vi "Read Msg Output.vi"(11 "TEMPLATE Msg Output in":refnum<class "TEMPLATE Msg Output.lvclass">) -> ()   [LabVIEW 2020, in "_Template.lvlib" / "Templates.lvlib" / "TEMPLATE jettl Msg.lvlib" / "TEMPLATE Msg Output.lvlib" / "TEMPLATE Msg Output.lvclass"]
uses:
  TEMPLATE Msg Output.lvclass
panel:
  # "This front panel should not be manipulated."
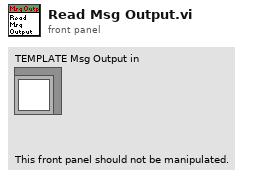
[diagram p1: front panel]
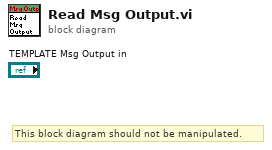
[diagram p0: block diagram]
diagram:
  # "This block diagram should not be manipulated."
